vi "Sequence Editor.vi"() -> ()   [LabVIEW 2013, in "Simple Sequence Tools - Editor.lvlib"]
uses:
  Simple Sequence Tools - Editor.lvlib
  Types/UI.PropertiesTypes.ctl
  Types/StateVariables.ctl
  Shared/Types/ChannelProperties.ctl
  Shared/Types/INI.Settings
  Shared/Simple Sequence Tools - Shared.lvlib
panel:
  in  "Sequence":i32[](listbox)
  in  "Iteration Information Channel":string(combo)
  in  "Iterations":u32=1 min=1
  in  "View":T1=enum."Sequence Properties"
  in  "Abort Channel":string(combo)
  in  "Step Information Channel":string(combo)
  out "Graph":waveform(dbl)[](graph)
  out "Path":path
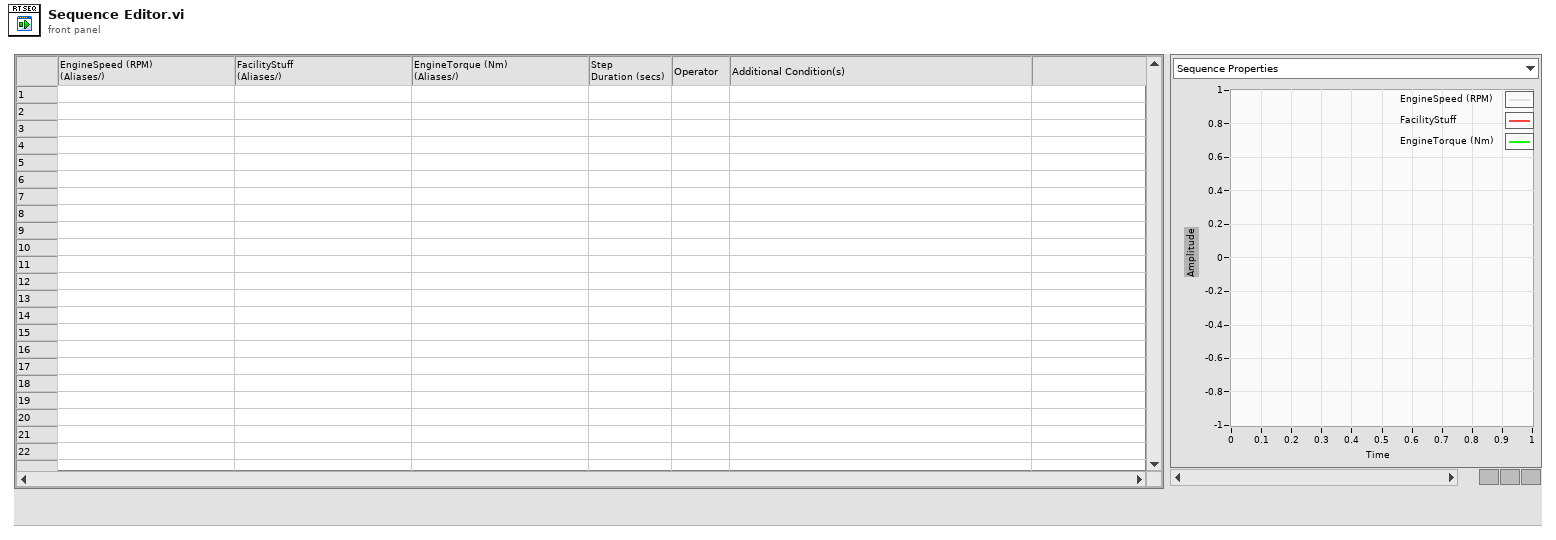
[diagram p1: front panel]
types:
  T1 = typedef "Simple Sequence Tools - Editor.lvlib/UI.PropertiesTypes.ctl" = enum8{"Step Properties", "Sequence Properties"}
  T2 = typedef "Simple Sequence Tools - Editor.lvlib/StateVariables.ctl" = cluster{"Aliases.All":T3[], "Aliases.Outputs":T3[], "UI.Sequence#ofColumns":i32, "SysDef.Path":path, "UI.SequenceRef":refnum<vi>, "UI.StepInformationRef":refnum<vi>, "UI.AbortRef":refnum<vi>, "UI.GraphRef":refnum<vi>, "UI.ViewRef":refnum<vi>, "UI.IterationsRef":refnum<vi>, "UI.IterationInformationRef":refnum<vi>, "INI.Settings":T4}
  T3 = typedef "Simple Sequence Tools - Shared.lvlib/ChannelProperties.ctl" = cluster{"Name":string, "NodePath":string, "ScaleUnits":string}
  T4 = typedef "Simple Sequence Tools - Shared.lvlib/INI.Settings" = cluster{"Build Location":path, "LoggingLocation":path}
  T5 = typedef "LVPoint32TypeDef.ctl" = cluster{"Horizontal":i32, "Vertical":i32}
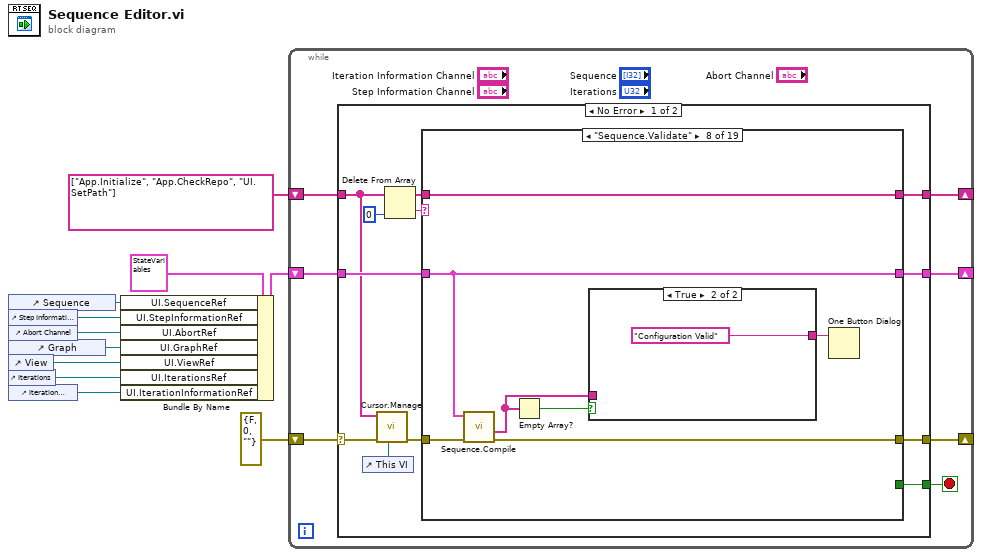
[diagram p0: block diagram]
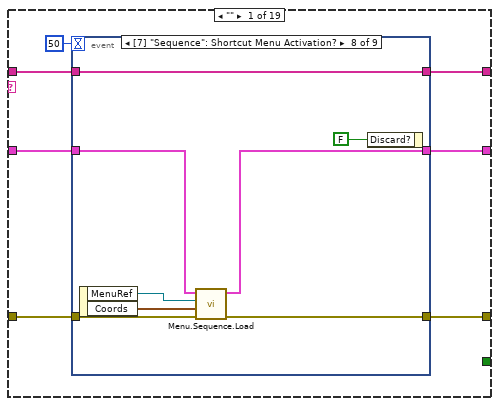
[diagram p2: hidden frame]
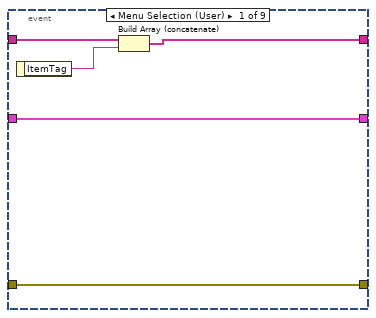
[diagram p3: hidden frame]
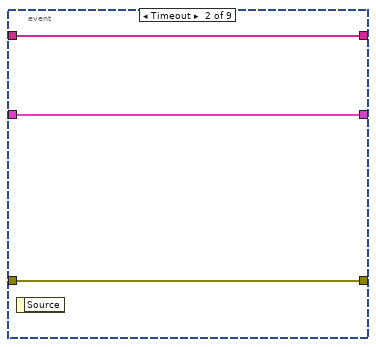
[diagram p4: hidden frame]
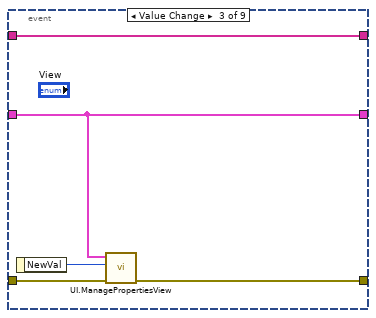
[diagram p5: hidden frame]
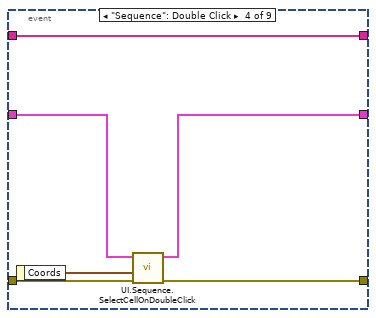
[diagram p6: hidden frame]
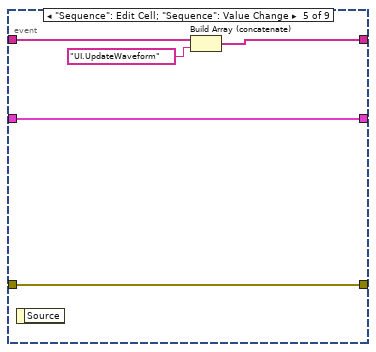
[diagram p7: hidden frame]
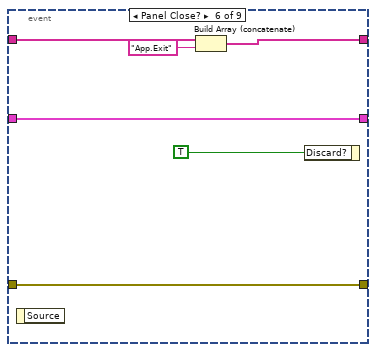
[diagram p8: hidden frame]
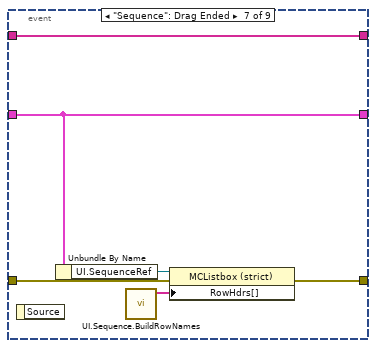
[diagram p9: hidden frame]
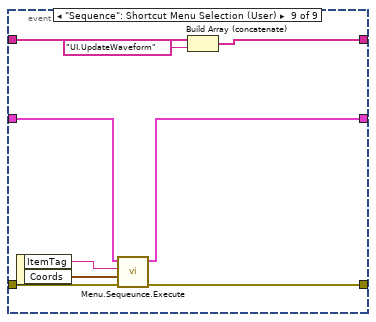
[diagram p10: hidden frame]
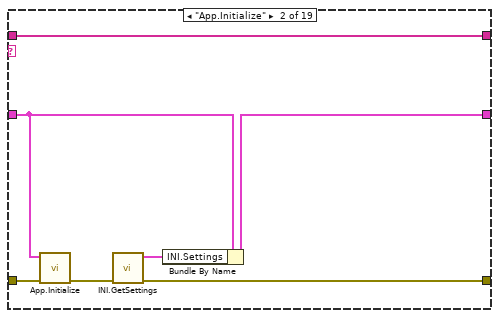
[diagram p11: hidden frame]
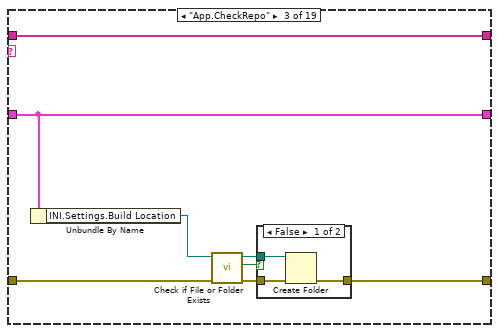
[diagram p12: hidden frame]
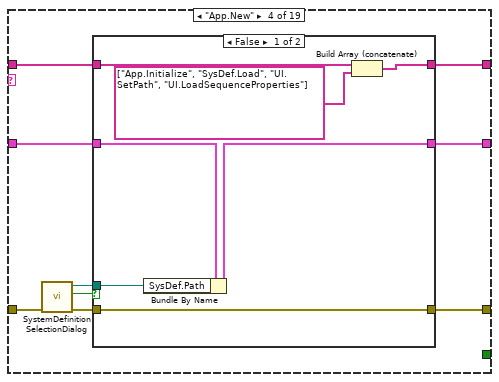
[diagram p14: hidden frame]
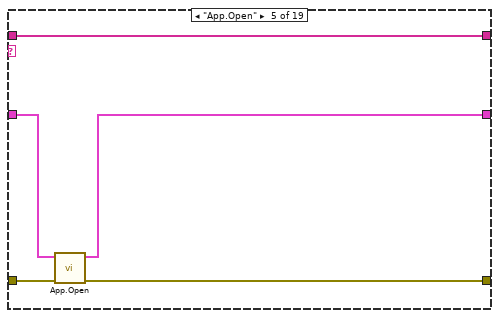
[diagram p16: hidden frame]
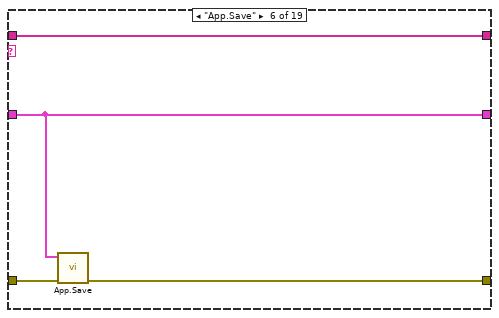
[diagram p17: hidden frame]
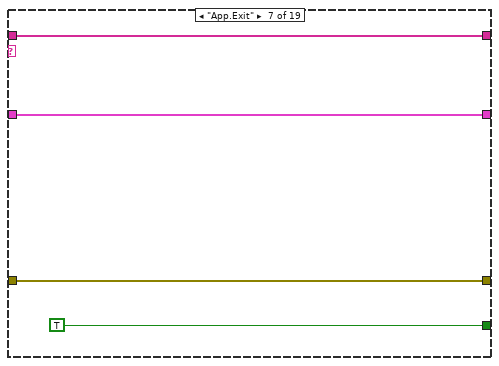
[diagram p18: hidden frame]
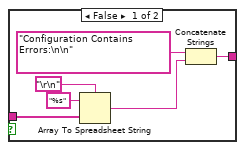
[diagram p19: hidden frame]
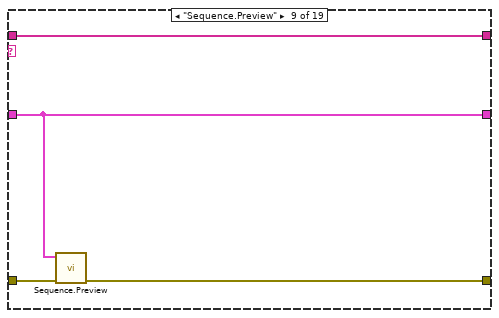
[diagram p20: hidden frame]
diagram:
  n1 = control-ref of="Sequence"() -> (w7:refnum<vi>)
  n2 = control-ref of="Step Information Channel"() -> (w6:refnum<vi>)
  n3 = control-ref of="Abort Channel"() -> (w5:refnum<vi>)
  n4 = control-ref of="Graph"() -> (w4:refnum<vi>)
  n5 = control-ref of="View"() -> (w3:refnum<vi>)
  n6 = control-ref of="Iterations"() -> (w2:refnum<vi>)
  n7 = control-ref of="Iteration Information Channel"() -> (w1:refnum<vi>)
  n8 = Bundle By Name(cluster=T2 {"Aliases.All"=[], "Aliases.Outputs"=[], "UI.Sequence#ofColumns"=0, "SysDef.Path"=path "", "UI.SequenceRef"=refnum, "UI.StepInformationRef"=refnum, "UI.AbortRef"=refnum, "UI.GraphRef"=refnum, "UI.ViewRef"=refnum, "UI.IterationsRef"=refnum, "UI.IterationInformationRef"=refnum, "INI.Settings"={"Build Location"=path "", "LoggingLocation"=path ""}}, "UI.SequenceRef"=w7, "UI.StepInformationRef"=w6, "UI.AbortRef"=w5, "UI.GraphRef"=w4, "UI.ViewRef"=w3, "UI.IterationsRef"=w2, "UI.IterationInformationRef"=w1) -> (w8:T2)
  n9 = while {
    shift-right: [w17] -> _
    shift-left: string[] ["App.Initialize", "App.CheckRepo", "UI.SetPath"] -> [w18]
    shift-right: [w15] -> _
    shift-left: w8 -> [w16]
    shift-right: [w13] -> _
    shift-left: errorcluster {"status"=FALSE, "code"=0, "source"=""} ("error constant") -> [w14]
    stop <- w12 stop-if-true
    n10 = case shown="No Error" w14 {
      selector: w14 -> [w22 w222]
      tunnel: w18 -> [w23 w225]
      tunnel: [w29 w225] -> w17
      tunnel: w16 -> [w27 w224]
      tunnel: [w26 w224] -> w15
      tunnel: [w25 w221] -> w13
      tunnel: [w24 _] -> w12
      frame No Error {
        n11 = control-ref of="This VI"() -> (w19:refnum<vi>)
        n12 = call "Cursor.Manage.vi"("VI reference (current VI)"=w19, "error in (no error)"=w22, "Cmd list"=w23) -> ("error out"=w21:errorcluster)  [unwired: 8 in]
        n13 = Delete From Array(array=w23, index=0) -> (deleted portion=w30:string, array with subset deleted=w28:string[])  [unwired: 1 in]
        n14 = case shown="\"Sequence.Validate\"" w30 {
          tunnel: [w34 w97 w105 w110 w133 w137 w141 w148 w159 w163 w164 w190 w194 w198 w203 w207 w213 w217 w220] -> w29
          tunnel: w28 -> [w33 w97 w105 w111 w133 w137 w141 w148 w159 w163 w165 w190 w194 w199 w203 w207 w213 w217 w220]
          tunnel: w27 -> [w36 w92 w104 w114 w130 w135 w140 w145 w158 w160 w168 w187 w193 w195 w200 w205 w209 w216 w219]
          tunnel: [w37 w91 w104 w112 w129 w135 w140 w145 w158 w160 w166 w186 w193 w195 w200 w205 w210 w216 w219] -> w26
          tunnel: [w31 w94 w99 w115 w131 w136 w139 w146 w156 w162 w169 w188 w191 w196 w201 w206 w211 w214 w218] -> w25
          tunnel: w21 -> [w32 w96 w102 w117 w132 w134 w139 w147 w157 w161 w171 w183 w192 w196 w202 w206 w208 w215 w218]
          tunnel: [_ _ _ _ _ _ TRUE _ _ _ _ _ _ _ _ _ _ _ _] -> w24
          frame "" {
            n15 = event shown="[7] \"Sequence\": Shortcut Menu Activation?" {
              selector: _ -> [_ _ _ _ _ _ _ _ _]
              dyn-events: _ -> [_ _ _ _ _ _ _ _ _]
              timeout: 50 -> [_ _ _ _ _ _ _ _ _]
              tunnel: [w39 w45 w50 w56 w58 w63 w73 w81 w83] -> w34
              tunnel: w33 -> [w41 w45 w50 w56 w61 w67 w73 w81 w90]
              tunnel: [w42 w44 w49 w51 w60 w66 w69 w77 w84] -> w37
              tunnel: w36 -> [w42 w44 w49 w52 w60 w66 w69 w76 w85]
              tunnel: [w40 w43 w46 w53 w59 w65 w70 w78 w86] -> w31
              tunnel: w32 -> [w40 w43 w48 w54 w59 w65 w71 w79 w87]
              event Menu Selection (User) {
                n16 = event-data() -> ("ItemTag"=w38:string)  [unwired: 1 in]
                n17 = Build Array (concatenate)(w41, w38) -> (w39:string[])
              }
              event Timeout {
                n18 = event-data() -> ()  [unwired: 1 in, 1 out]
              }
              event Value Change {
                n19 = event-data() -> ("NewVal"=w47:T1)  [unwired: 1 in]
                n20 = call "UI.ManagePropertiesView.vi"("error in (no error)"=w48, "NewVal"=w47, "State Variables"=w49) -> ("error out"=w46:errorcluster)  [unwired: 8 in]
              }
              event "Sequence": Double Click {
                n21 = event-data() -> ("Coords"=w55:T5)  [unwired: 1 in]
                n22 = call "UI.Sequence.SelectCellOnDoubleClick.vi"("error in (no error)"=w54, "Coords"=w55, "State Variables"=w52) -> ("error out"=w53:errorcluster, "State Variables out"=w51:T2)  [unwired: 7 in]
              }
              event "Sequence": Edit Cell; "Sequence": Value Change {
                n23 = event-data() -> ()  [unwired: 1 in, 1 out]
                n24 = Build Array (concatenate)(w61, "UI.UpdateWaveform" ("message")) -> (w58:string[])
              }
              event Panel Close? {
                n25 = event-data() -> ()  [unwired: 1 in, 1 out]
                n26 = Build Array (concatenate)(w67, "App.Exit") -> (w63:string[])
                n27 = event-data("Discard?"=TRUE) -> ()  [unwired: 1 in, 1 out]
              }
              event "Sequence": Drag Ended {
                n28 = event-data() -> ()  [unwired: 1 in, 1 out]
                n29 = Unbundle By Name(w69) -> ("UI.SequenceRef"=w68:refnum<vi>)
                n30 = call "UI.Sequence.BuildRowNames.vi"() -> ("Row Headings"=w72:string[])  [unwired: 11 in]
                n31 = property class="MCListbox (strict)"(reference=w68, error in=w71, "RowHdrs[]"=w72) -> (error out=w70:errorcluster)  [unwired: 1 out]
              }
              event "Sequence": Shortcut Menu Activation? {
                n32 = event-data() -> ("MenuRef"=w74:refnum<k9>, "Coords"=w75:T5)  [unwired: 1 in]
                n33 = call "Menu.Sequence.Load.vi"("error in (no error)"=w79, "Coords"=w75, "MenuRef"=w74, "State Variables"=w76) -> ("error out"=w78:errorcluster, "State Variables out"=w77:T2)  [unwired: 6 in]
                n34 = event-data("Discard?"=FALSE) -> ()  [unwired: 1 in, 1 out]
              }
              event "Sequence": Shortcut Menu Selection (User) {
                n35 = event-data() -> ("ItemTag"=w89:string, "Coords"=w88:T5)  [unwired: 1 in]
                n36 = call "Menu.Sequeunce.Execute.vi"("error in (no error)"=w87, "Coords"=w88, "ItemPath"=w89, "State Variables"=w85) -> ("error out"=w86:errorcluster, "State Variables out"=w84:T2)  [unwired: 6 in]
                n37 = Build Array (concatenate)(w90, "UI.UpdateWaveform" ("message")) -> (w83:string[])
              }
            }
          }
          frame "App.Initialize" {
            n38 = call "App.Initialize.vi"("error in (no error)"=w96, "Start Variables"=w92) -> ("error out"=w95:errorcluster)  [unwired: 9 in]
            n39 = call "INI.GetSettings.vi"("error in (no error)"=w95) -> ("error out"=w94:errorcluster, "INI.Settings"=w93:T4)  [unwired: 9 in]
            n40 = Bundle By Name(cluster=w92, "INI.Settings"=w93) -> (w91:T2)
          }
          frame "App.CheckRepo" {
            n41 = Unbundle By Name(w104) -> ("INI.Settings.Build Location"=w103:path)
            n42 = call <vilib>:"Check if File or Folder Exists.vi"("error in (no error)"=w102, "path"=w103) -> ("error out"=w100:errorcluster, "file or folder exists?"=w98:bool, "dup path"=w101:path)  [unwired: 7 in]
            n43 = case shown="False" w98 {
              tunnel: w101 -> [w108 _]
              tunnel: w100 -> [w107 w109]
              tunnel: [w106 w109] -> w99
              frame False {
                n44 = Create Folder(path (use dialog)=w108, error in=w107) -> (error out=w106:errorcluster)  [unwired: 1 in, 2 out]
              }
              frame True {
              }
            }
          }
          frame "App.New" {
            n45 = call "SystemDefinitionSelectionDialog.vi"("error in (no error)"=w117) -> ("error out"=w118:errorcluster, "cancelled"=w116:bool, "selected path"=w113:path)  [unwired: 8 in]
            n46 = case shown="False" w116 {
              tunnel: w118 -> [w125 w127]
              tunnel: [w125 w127] -> w115
              tunnel: w114 -> [w124 w128]
              tunnel: [w123 w128] -> w112
              tunnel: w113 -> [w122 _]
              tunnel: [w121 w126] -> w110
              tunnel: w111 -> [w119 w126]
              frame False {
                n47 = Bundle By Name(cluster=w124, "SysDef.Path"=w122) -> (w123:T2)
                n48 = Build Array (concatenate)(w119, string[] ["App.Initialize", "SysDef.Load", "UI.SetPath", "UI.LoadSequenceProperties"]) -> (w121:string[])
              }
              frame True {
              }
            }
          }
          frame "App.Open" {
            n49 = call "App.Open.vi"("error in (no error)"=w132, "State Variables"=w130) -> ("error out"=w131:errorcluster, "State Variables out"=w129:T2)  [unwired: 8 in]
          }
          frame "App.Save" {
            n50 = call "App.Save.vi"("error in (no error)"=w134, "State Variables"=w135) -> ("error out"=w136:errorcluster)  [unwired: 9 in]
          }
          frame "App.Exit" {
          }
          frame "Sequence.Validate" {
            n51 = call "Sequence.Compile.vi"("error in (no error)"=w147, "State Variables"=w145) -> ("error out"=w146:errorcluster, "Warnings"=w142:string[])  [unwired: 7 in, 1 out]
            n52 = Empty Array?(array=w142) -> (empty?=w144:bool)
            n53 = case shown="True" w144 {
              tunnel: [w152 "Configuration Valid"] -> w143
              tunnel: w142 -> [w153 _]
              frame False {
                n54 = Array To Spreadsheet String(delimiter (Tab)="\r\n", array=w153, 3:"%s" ("format string")) -> (spreadsheet string=w151:string)
                n55 = Concatenate Strings("Configuration Contains Errors:\n\n", w151) -> (w152:string)
              }
              frame True {
              }
            }
            n56 = One Button Dialog(message=w143) -> ()  [unwired: 1 in, 1 out]
          }
          frame "Sequence.Preview" {
            n57 = call "Sequence.Preview.vi"("error in (no error)"=w157, "State Variables"=w158) -> ("error out"=w156:errorcluster)  [unwired: 9 in]
          }
          frame "Sequence.Build" {
            n58 = call "Sequence.Build.vi"("error in (no error)"=w161, "State Variables"=w160) -> ("error out"=w162:errorcluster)  [unwired: 9 in]
          }
          frame "SysDef.New" {
            n59 = call "SystemDefinitionSelectionDialog.vi"("error in (no error)"=w171) -> ("error out"=w172:errorcluster, "cancelled"=w170:bool, "selected path"=w167:path)  [unwired: 8 in]
            n60 = case shown="False" w170 {
              tunnel: w172 -> [w179 w181]
              tunnel: [w179 w181] -> w169
              tunnel: w168 -> [w178 w182]
              tunnel: [w177 w182] -> w166
              tunnel: w167 -> [w176 _]
              tunnel: [w175 w180] -> w164
              tunnel: w165 -> [w173 w180]
              frame False {
                n61 = Bundle By Name(cluster=w178, "SysDef.Path"=w176) -> (w177:T2)
                n62 = Build Array (concatenate)(w173, string[] ["SysDef.Load", "UI.SetPath", "UI.LoadSequenceProperties"]) -> (w175:string[])
              }
              frame True {
              }
            }
          }
          frame "SysDef.Load" {
            n63 = Unbundle By Name(w187) -> ("SysDef.Path"=w189:path)
            n64 = call "LoadSystemDefinition.vi"("error in (no error)"=w183, "SysDef.Path"=w189) -> ("error out"=w188:errorcluster, "Aliases.Outputs"=w184:T3[], "Aliases.All"=w185:T3[])  [unwired: 7 in]
            n65 = Bundle By Name(cluster=w187, "Aliases.All"=w185, "Aliases.Outputs"=w184) -> (w186:T2)
          }
          frame "SysDef.Edit" {
            n66 = call "SysDef.Edit.vi"("error in (no error)"=w192, "State Variables"=w193) -> ("error out"=w191:errorcluster)  [unwired: 9 in]
          }
          frame "SysDef.Refresh" {
            n67 = Build Array (concatenate)(w199, string[] ["SysDef.Load", "UI.SetPath", "UI.LoadSequenceProperties"]) -> (w198:string[])
          }
          frame "Steps.GenerateMultiple" {
            n68 = call "Dialog.MassStepGeneration.vi"("error in (no error)"=w202, "State Variables"=w200) -> ("error out"=w201:errorcluster)  [unwired: 9 in]
          }
          frame "UI.SetPath" {
            n69 = Unbundle By Name(w205) -> ("SysDef.Path"=→"Path":path)
          }
          frame "UI.UpdateWaveform" {
            n70 = call "UI.UpdateWaveform.vi"("error in (no error)"=w208, "State Variables"=w209) -> ("error out"=w211:errorcluster, "Wavefrom"=→"Graph":waveform(dbl)[], "State Variables out"=w210:T2)  [unwired: 7 in]
          }
          frame "UI.LoadSequenceProperties" {
            n71 = call "UI.LoadComboBoxes.vi"("error in (no error)"=w215, "State Variables"=w216) -> ("error out"=w214:errorcluster)  [unwired: 9 in]
          }
          frame Default {
          }
        }
      }
      frame Error {
        n72 = call <vilib>:"Simple Error Handler.vi"("error in (no error)"=w222) -> ("error out"=w223:errorcluster)  [unwired: 4 in, 4 out]
        n73 = call <vilib>:"Clear Errors.vi"("error in (no error)"=w223) -> ("error out"=w221:errorcluster)  [unwired: 6 in]
      }
    }
  }
